vi "girpcutil_RpcValue_WriteToString.vi"(8 "Fehler (Eingang, kein Fehler)":errorcluster, 10 "value":i32, 11 "girpcutil_params":T1) -> (0 "Fehler (Ausgang)":errorcluster)   [LabVIEW 2016]
uses:
  girpcutil_params.ctl
panel:
  out "size of rpc value string":u32
  out "string":string
  out "errMsgLen":i32
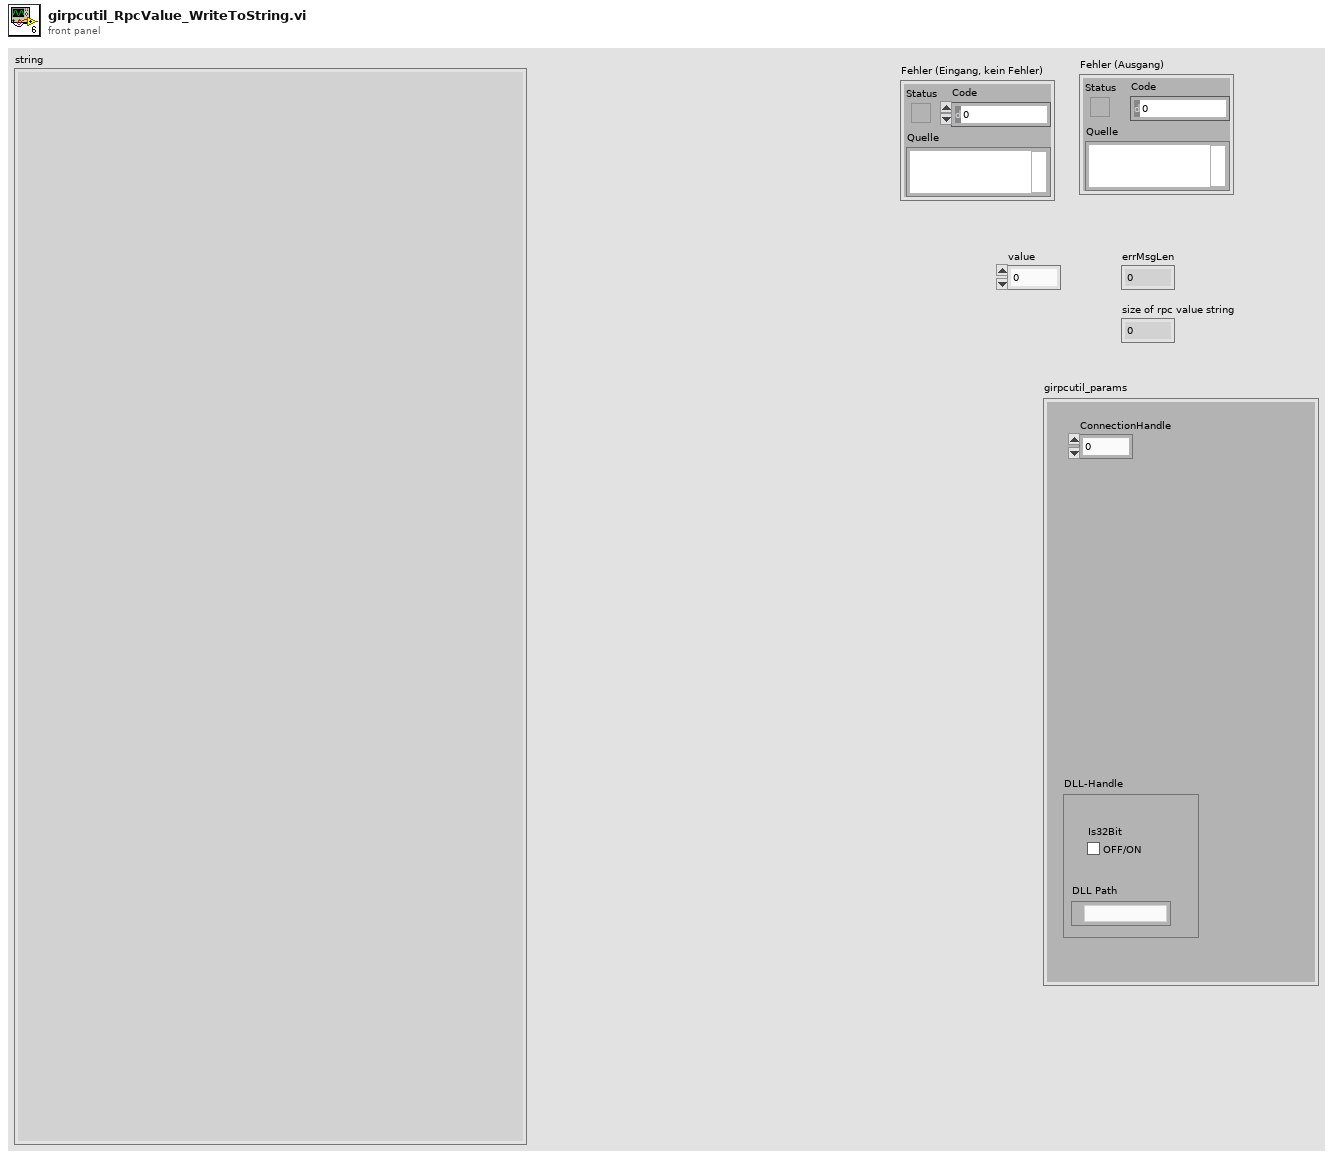
[diagram p1: front panel]
types:
  T1 = typedef "girpcutil_params.ctl" = cluster{"ConnectionHandle":i32, "DLL-Handle":cluster{"DLL Path":path, "Is32Bit":bool}}
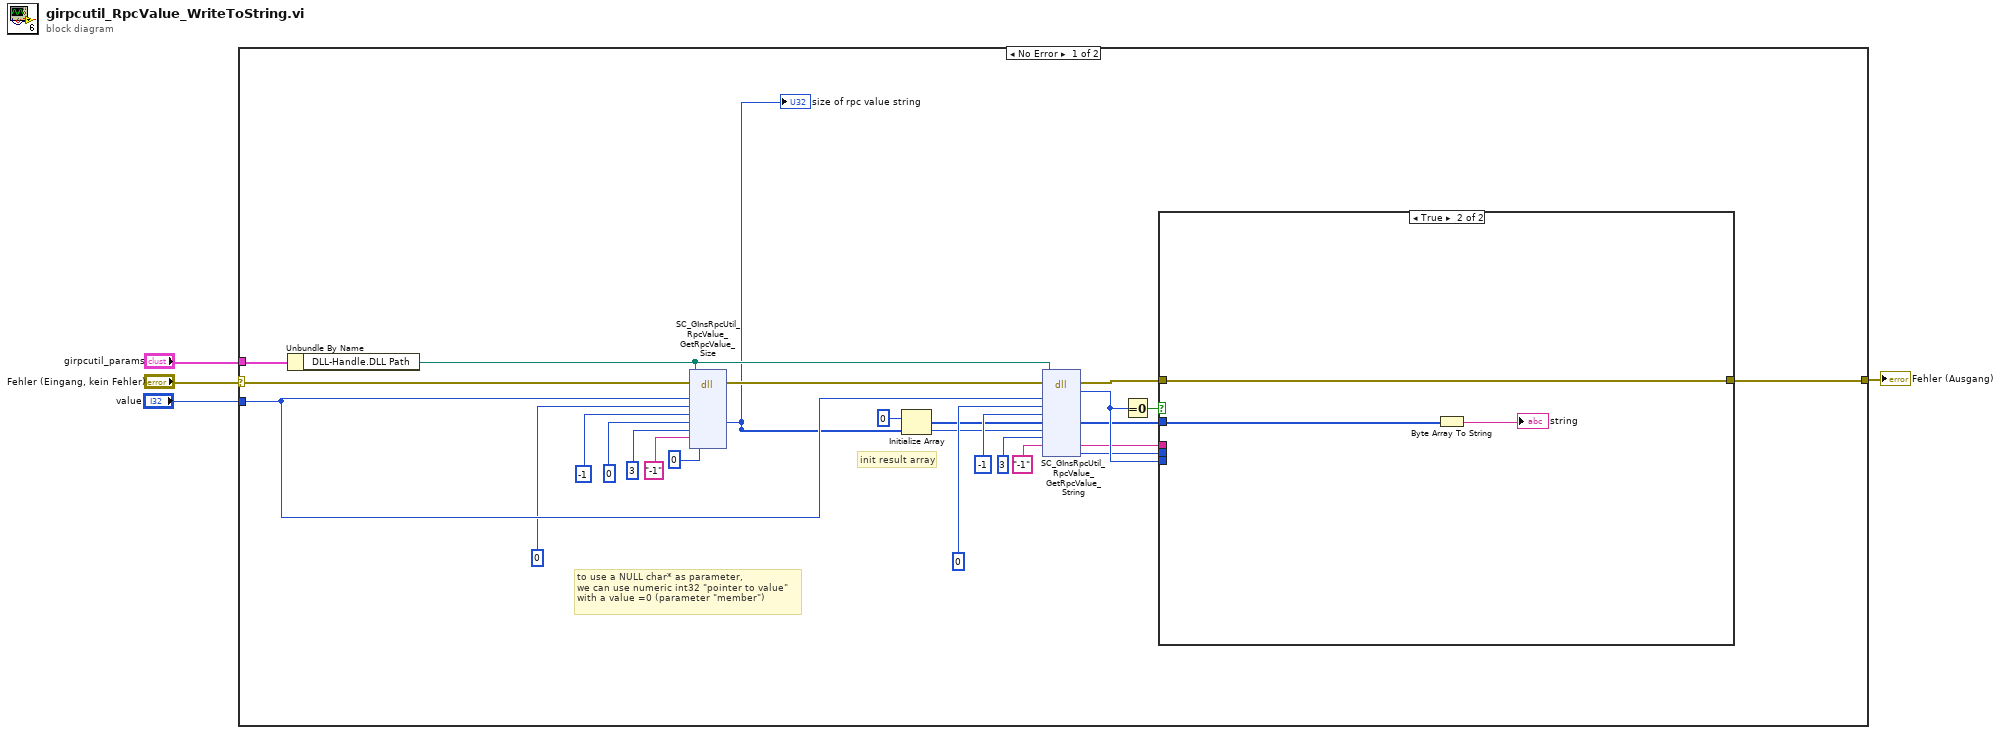
[diagram p0: block diagram]
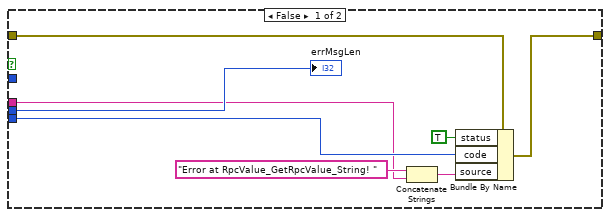
[diagram p2: hidden frame]
diagram:
  n1 = case shown="No Error" "Fehler (Eingang, kein Fehler)" {
    selector: "Fehler (Eingang, kein Fehler)" -> [w17 w41]
    tunnel: "girpcutil_params" -> [w29 _]
    tunnel: "value" -> [w14 _]
    tunnel: [w21 w41] -> w1
    frame No Error {
      # "init result array"
      # "to use a NULL char* as parameter, \nwe can use numeric int32 \"pointer to value\"\nwith a value =0 (parameter \"member\")"
      n2 = Unbundle By Name(w29) -> ("DLL-Handle.DLL Path"=w16:path)
      n3 = dll-call lib="?" fn="SC_GInsRpcUtil_RpcValue_GetRpcValue_Size"(path in=w16, error in=w17, "value"=w14, "member"=0, "index"=-1, "size"=u32 0, "tagSet"=u32 3, "errMsg"="-1", "errMsgLen"=0) -> (error out=w15:errorcluster, "size"=w6:u32)  [unwired: 8 in, 1 out]
      "size of rpc value string" <- w6
      n4 = Initialize Array(u8 0, w6) -> (w7:u8[])
      n5 = dll-call lib="?" fn="SC_GInsRpcUtil_RpcValue_GetRpcValue_String"(path in=w16, error in=w15, "value"=w14, "member"=0, "index"=-1, "result"=w7, "resultLen"=w6, "tagSet"=u32 3, "errMsg"="-1" ("result")) -> (error out=w26:errorcluster, "Rückgabewert"=w24:i32, "result"=w20:u8[], "errMsg"=w22:string, "errMsgLen"=w23:i32)  [unwired: 7 in, 1 out]
      n6 = Equal To 0?(x=w24) -> (x = 0?=w25:bool)
      n7 = case shown="True" w25 {
        tunnel: w26 -> [w33 w40]
        tunnel: [w32 w40] -> w21
        tunnel: w22 -> [w30 _]
        tunnel: w23 -> [w34 _]
        tunnel: w24 -> [w31 _]
        tunnel: w20 -> [_ w39]
        frame False {
          n8 = Concatenate Strings("Error at RpcValue_GetRpcValue_String! " ("source"), w30) -> (w36:string)
          n9 = Bundle By Name(cluster=w33, "status"=TRUE, "code"=w31, "source"=w36) -> (w32:errorcluster)
          "errMsgLen" <- w34
        }
        frame True {
          n10 = Byte Array To String(unsigned byte array=w39) -> (string=→"string":string)
        }
      }
    }
    frame Error {
    }
  }
  "Fehler (Ausgang)" <- w1
